vi "Check Serial Parsing --Unit Test.vi"   [LabVIEW 2021]
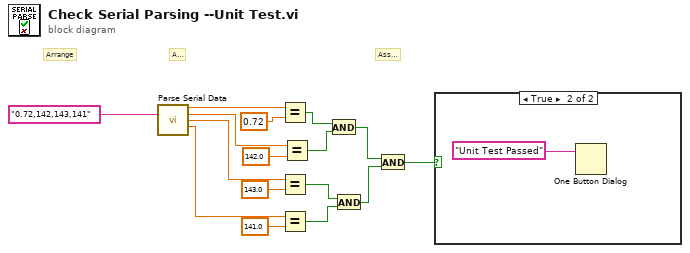
[diagram p0: block diagram]
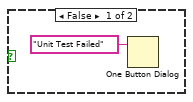
[diagram p2: hidden frame]
diagram:
  # "Assert"
  # "Act"
  # "Arrange"
  n1 = call "Parse Serial Data.vi"("Serial String"="0.72,142,143,141") -> ("Pressure"=w15:dbl, "Temp1"=w13:dbl, "Temp2"=w11:dbl, "Temp3"=w9:dbl)  [unwired: 10 in, 1 out]
  n2 = Equal?(x=w15, y=0.72) -> (x = y?=w7:bool)
  n3 = Equal?(x=w11, y=143.0) -> (x = y?=w5:bool)
  n4 = Equal?(x=w9, y=141.0) -> (x = y?=w4:bool)
  n5 = Equal?(x=w13, y=142.0) -> (x = y?=w6:bool)
  n6 = And(x=w7, y=w6) -> (x .and. y?=w3:bool)
  n7 = And(x=w5, y=w4) -> (x .and. y?=w2:bool)
  n8 = And(x=w3, y=w2) -> (x .and. y?=w1:bool)
  n9 = case shown="True" w1 {
    frame False {
      n10 = One Button Dialog(message="Unit Test Failed") -> ()  [unwired: 1 in, 1 out]
    }
    frame True {
      n11 = One Button Dialog(message="Unit Test Passed") -> ()  [unwired: 1 in, 1 out]
    }
  }
